vi "test图层(1)-原版.vi"() -> ()   [LabVIEW 2018]
doc: "This example demonstrates the use of binary morphological reconstruction in the particle analysis. The example allows you to keep the particles completely inside the ROI, completely outside the ROI or on the ROI."
uses:
  <vilib>/vision/NI_Vision_Development_Module.lvlib
panel:
  out "框&图层计数":dbl
  in  "Operation":T1(ring)
  out "Reconstructed Image":T2(plugin-control)
  out "Image":T2(plugin-control)
  in  "Stop":bool
  # "Overview: Demonstrate the use of the Binary Morphology Reconstruction feature of Vision Development Module.\nRequirements: Vision Development Module.\nInstructions:\n1. Run the VI.\n2. Select the ROI in which you want to filter the objects. Press the <Ctrl> key to select multiple ROIs. \n3. Choose the required \"Operation\".\n  - Inner particles: Keeps all the particles completely inside the ROI.\n  - Outer particles: Keeps the particles completely outside the ROI.\n  - Boundary particles: Keeps the particles which are touching the boundary."
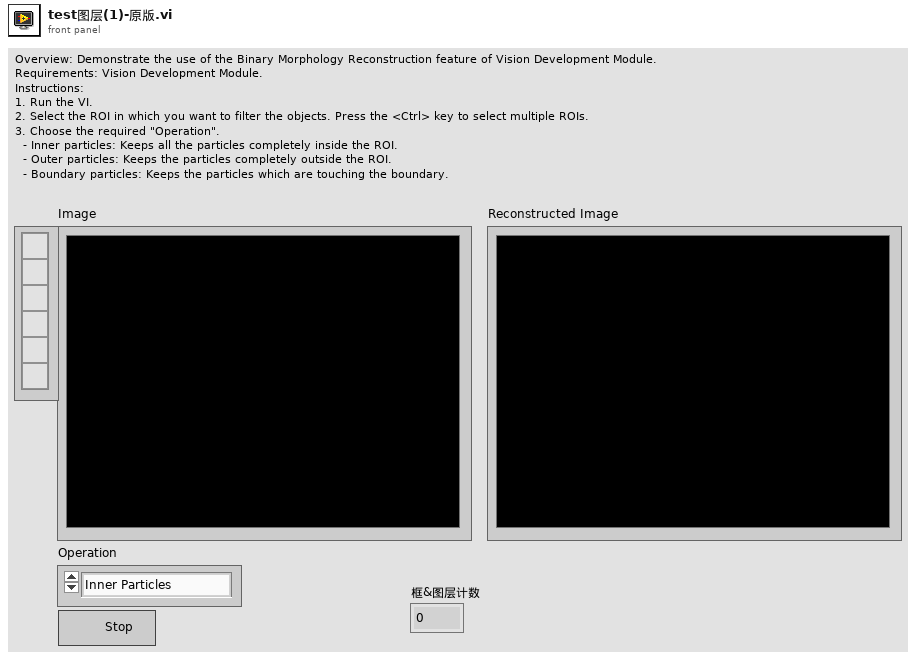
[diagram p1: front panel]
types:
  T1 = enum16{"Inner Particles", "Outer Particles", "Boundary Particles", "overlay rectangle"}
  T2 = typedef "IMAQ Image.ctl" = refnum<image>
  T3 = typedef "Image Type" = u32
  T4 = cluster{"Global Rectangle":i32[], "Contours":cluster{"Contour Type":u32, "ROI Type":u32, "Points":i32[]}[]}
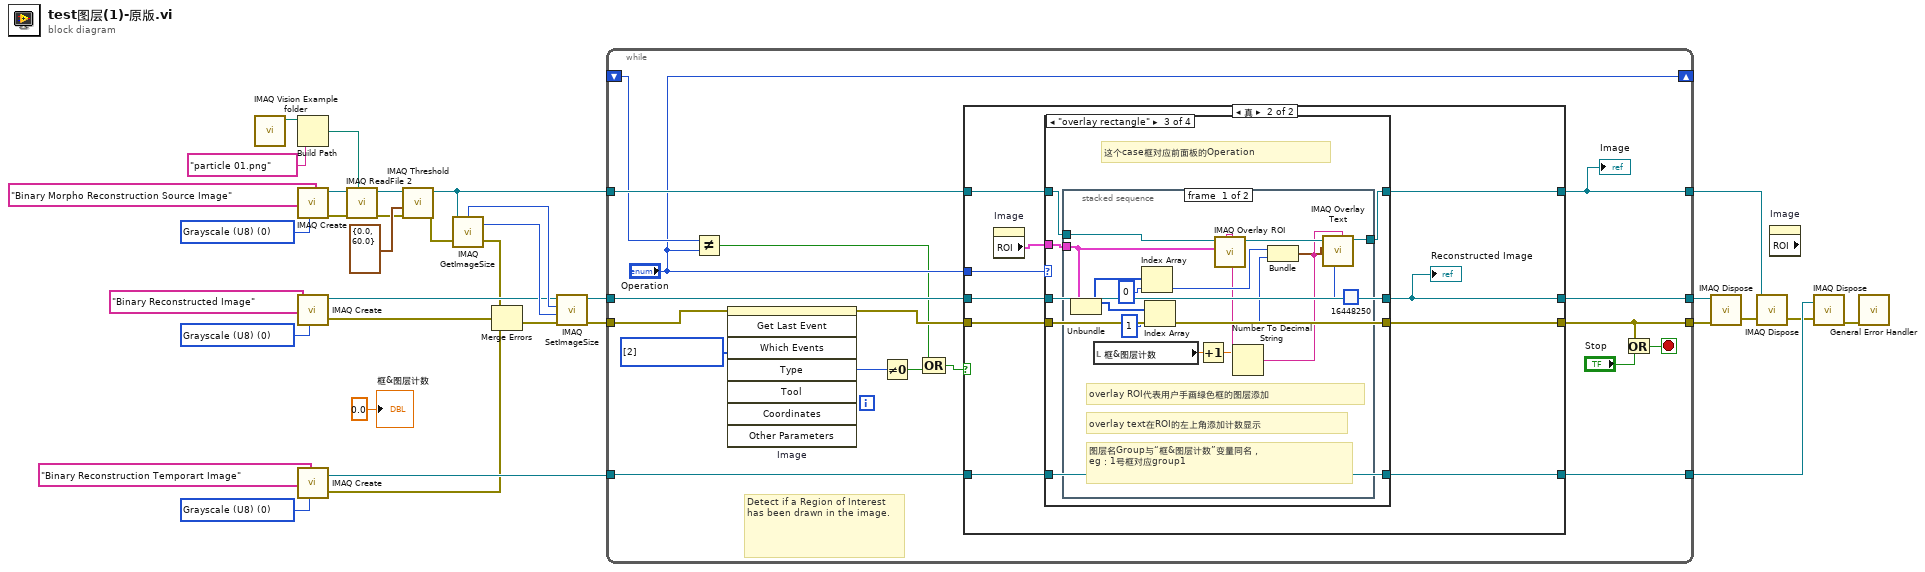
[diagram p0: block diagram]
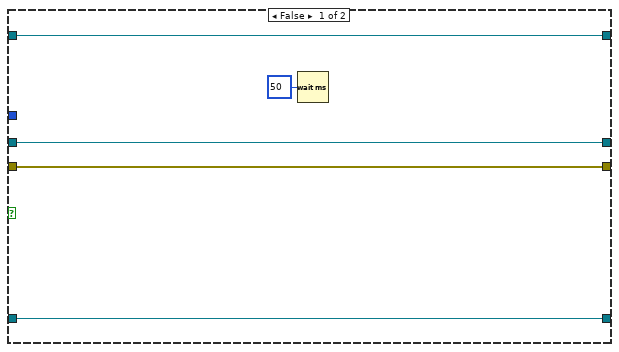
[diagram p2: hidden frame]
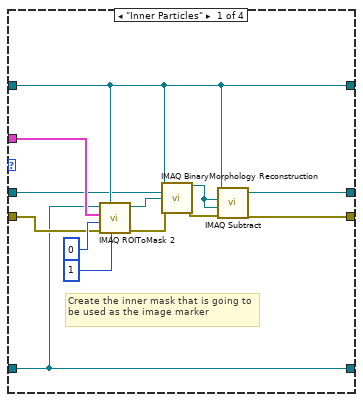
[diagram p3: hidden frame]
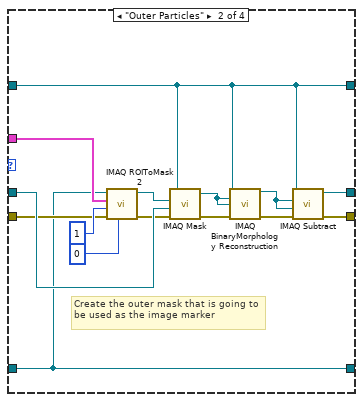
[diagram p4: hidden frame]
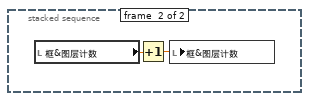
[diagram p5: hidden frame]
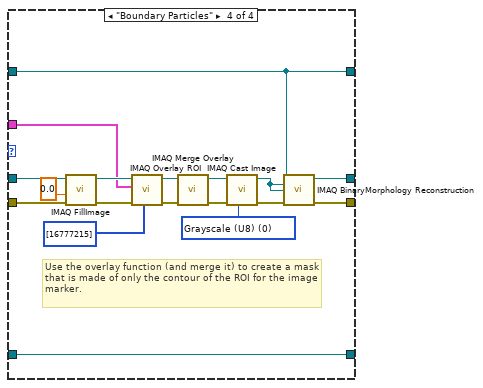
[diagram p6: hidden frame]
diagram:
  w24 = T3 0 items=["Grayscale (U8)", "Grayscale (I16)", "Grayscale (SGL)", "Complex (CSG)", "RGB (U32)", "HSL (U32)", "RGB (U64)", "Grayscale (U16)"] ("Image Type")
  w26 = T3 0 items=["Grayscale (U8)", "Grayscale (I16)", "Grayscale (SGL)", "Complex (CSG)", "RGB (U32)", "HSL (U32)", "RGB (U64)", "Grayscale (U16)"] ("Image Type")
  w27 = T3 0 items=["Grayscale (U8)", "Grayscale (I16)", "Grayscale (SGL)", "Complex (CSG)", "RGB (U32)", "HSL (U32)", "RGB (U64)", "Grayscale (U16)"] ("Image Type")
  n1 = call "IMAQ Vision Example folder.vi"() -> ("Example Image Path"=w33:path)  [unwired: 11 in]
  n2 = Build Path(base path=w33, name or relative path="particle 01.png") -> (appended path=w3:path)
  n3 = call "IMAQ Create"("Image Name"="Binary Morpho Reconstruction Source Image", "Image Type"=w26) -> ("New Image"=w30:T2, "error out"=w16:errorcluster)  [unwired: 2 in, 1 out]
  n4 = call "IMAQ Create"("Image Name"="Binary Reconstructed Image", "Image Type"=w27) -> ("New Image"=w20:T2, "error out"=w13:errorcluster)  [unwired: 2 in, 1 out]
  n5 = call "IMAQ Create"("Image Name"="Binary Reconstruction Temporart Image", "Image Type"=w24) -> ("New Image"=w21:T2, "error out"=w12:errorcluster)  [unwired: 2 in, 1 out]
  n6 = call "IMAQ ReadFile 2"("File Path"=w3, "error in (no error)"=w16, "Image"=w30) -> ("error out"=w15:errorcluster, "Image Out"=w18:T2)  [unwired: 4 in, 3 out]
  n7 = call "IMAQ Threshold"("error in (no error)"=w15, "Range"=cluster{"Lower value":sgl, "Upper value":sgl} {"Lower value"=0.0, "Upper value"=60.0}, "Image Src"=w18) -> ("error out"=w14:errorcluster, "Image Dst Out"=w2:T2)  [unwired: 3 in, 4 out]
  n8 = call "IMAQ GetImageSize"("Image"=w2, "error in (no error)"=w14) -> ("Y Resolution"=w22:i32, "X Resolution"=w23:i32, "error out"=w9:errorcluster)  [unwired: 2 out]
  n9 = Merge Errors(w9, w13, w12) -> (w11:errorcluster)
  n10 = call "IMAQ SetImageSize"("error in (no error)"=w11, "Y Resolution"=w22, "X Resolution"=w23, "Image"=w20) -> ("error out"=w10:errorcluster, "Image Out"=w19:T2)  [unwired: 1 out]
  n11 = while {
    tunnel: w2 -> [w52]
    tunnel: w19 -> [w51]
    tunnel: [w50] -> w29
    tunnel: [w35] -> w28
    tunnel: w21 -> [w49]
    shift-right: ["Operation"] -> _
    shift-left: _ -> [w48]
    tunnel: w10 -> [w44]
    tunnel: [w38] -> w7
    tunnel: [w42] -> w8
    stop <- w36 stop-if-true
    w45 = i32[] [2] items=["No Event"=0, "Click Event"=1, "Draw Event"=2, "Size Event"=4, "Scroll Event"=5, "Double Click Event"=8] ("Which Events")
    # "Detect if a Region of Interest has been drawn in the image."
    n12 = Not Equal?(x=w48, y="Operation") -> (x != y?=w41:bool)
    n13 = invoke on="Image" class="ImageControl" method="Get Last Event"(error in=w44, "Which Events"=w45) -> (error out=w43:errorcluster, "Type"=w46:i32)  [unwired: 6 in, 6 out]
    n14 = Not Equal To 0?(x=w46) -> (x != 0?=w40:bool)
    n15 = Compound Arithmetic op=OR(w41, w40) -> (w39:bool)
    n16 = case shown="真" w39 {
      tunnel: w52 -> [w57 w67]
      tunnel: w51 -> [w56 w66]
      tunnel: [w56 w65] -> w50
      tunnel: [w57 w64] -> w35
      tunnel: w49 -> [w54 w59]
      tunnel: "Operation" -> [_ w62]
      tunnel: w43 -> [w55 w61]
      tunnel: [w55 w60] -> w38
      tunnel: [w54 w58] -> w42
      frame False {
        n17 = Wait (ms)(milliseconds to wait=u32 50) -> ()  [unwired: 1 out]
      }
      frame True {
        n18 = property on="Image" class="ImageControl"() -> ("ROI"=w63:T4)  [unwired: 2 in, 2 out]
        n19 = case shown="\"overlay rectangle\"" w62 {
          tunnel: w67 -> [w75 w87 w98 w132]
          tunnel: w66 -> [w73 w88 w101 w124]
          tunnel: w59 -> [w68 w81 w99 w133]
          tunnel: [w77 w90 w101 w135] -> w65
          tunnel: w63 -> [w76 w89 w96 w125]
          tunnel: [w75 w87 w97 w132] -> w64
          tunnel: w61 -> [w72 w86 w100 w123]
          tunnel: [w69 w82 w100 w134] -> w60
          tunnel: [w68 w81 w99 w133] -> w58
          frame "Inner Particles" {
            # "Create the inner mask that is going to be used as the image marker"
            n20 = call "IMAQ ROIToMask 2"("Background Value (0)"=1, "Image Model"=w75, "error in (no error)"=w72, "Filling Value (255)"=0, "ROI Descriptor"=w76, "Image"=w68) -> ("error out"=w71:errorcluster, "Image Out"=w74:T2)  [unwired: 4 out]
            n21 = call "IMAQ BinaryMorphology Reconstruction"("Image Src"=w75, "Image Dst"=w73, "Image Marker"=w74, "error in (no error)"=w71) -> ("Image Dst Out"=w78:T2, "error out"=w70:errorcluster)  [unwired: 4 in, 6 out]
            n22 = call "IMAQ Subtract"("Image Src A"=w75, "Image Dst"=w78, "Image Src B"=w78, "error in (no error)"=w70) -> ("Image Dst Out"=w77:T2, "error out"=w69:errorcluster)  [unwired: 1 in, 2 out]
          }
          frame "Outer Particles" {
            # "Create the outer mask that is going to be used as the image marker"
            n23 = call "IMAQ ROIToMask 2"("Background Value (0)"=0, "error in (no error)"=w86, "Filling Value (255)"=1, "ROI Descriptor"=w89, "Image"=w81) -> ("error out"=w85:errorcluster, "Image Out"=w93:T2)  [unwired: 1 in, 4 out]
            n24 = call "IMAQ Mask"("error in (no error)"=w85, "Image Dst"=w88, "Image Mask"=w93, "Image Src"=w87) -> ("error out"=w84:errorcluster, "Image Dst Out"=w92:T2)  [unwired: 1 out]
            n25 = call "IMAQ BinaryMorphology Reconstruction"("Image Src"=w87, "Image Dst"=w92, "Image Marker"=w92, "error in (no error)"=w84) -> ("Image Dst Out"=w91:T2, "error out"=w83:errorcluster)  [unwired: 4 in, 6 out]
            n26 = call "IMAQ Subtract"("Image Src A"=w87, "Image Dst"=w91, "Image Src B"=w91, "error in (no error)"=w83) -> ("Image Dst Out"=w90:T2, "error out"=w82:errorcluster)  [unwired: 1 in, 2 out]
          }
          frame "overlay rectangle" {
            # "这个case框对应前面板的Operation"
            n27 = stacked-sequence {
              tunnel: w98 -> [w115 _]
              tunnel: [w113 _] -> w97
              tunnel: w96 -> [w112 _]
              frame #0 {
                # "图层名Group与“框&图层计数”变量同名，\neg：1号框对应group1"
                # "overlay text在ROI的左上角添加计数显示"
                # "overlay ROI代表用户手画绿色框的图层添加"
                n28 = Unbundle(w112) -> ("Global Rectangle"=w109:i32[])  [unwired: 1 out]
                n29 = local read "框&图层计数"() -> (w104:dbl)
                n30 = Index Array(array=w109, index=0 ("索引")) -> (element=w108:i32)
                n31 = Index Array(array=w109, index=1 ("索引")) -> (element=w107:i32)
                n32 = Increment(x=w104) -> (x+1=w102:dbl)
                n33 = Number To Decimal String(number=w102) -> (decimal integer string=w103:string)  [unwired: 1 in]
                n34 = call "IMAQ Overlay ROI"("Group"=w103, "ROI Descriptor"=w112, "Image"=w115) -> ("Image Out"=w114:T2)  [unwired: 7 in, 1 out]
                n35 = Bundle(w108, w107) -> (w106:cluster{i32, i32})  [unwired: 1 in]
                n36 = call "IMAQ Overlay Text"("Group"=w103, "Text Color (black)"=u32 16448250, "String"=w103, "Origin"=w106, "Image"=w114) -> ("Image Out"=w113:T2)  [unwired: 5 in, 1 out]
              }
              frame #1 {
                n37 = local read "框&图层计数"() -> (w117:dbl)
                n38 = Increment(x=w117) -> (x+1=w116:dbl)
                n39 = local write "框&图层计数"(w116) -> ()
              }
            }
          }
          frame "Boundary Particles" {
            w127 = T3 0 items=["Grayscale (U8)", "Grayscale (I16)", "Grayscale (SGL)", "Complex (CSG)", "RGB (U32)", "HSL (U32)", "RGB (U64)", "Grayscale (U16)"] ("Image Type")
            # "Use the overlay function (and merge it) to create a mask that is made of only the contour of the ROI for the image marker."
            n40 = call "IMAQ FillImage"("error in (no error)"=w123, "Pixel Value (U8, U16, I16, Float)"=sgl 0.0, "Image"=w124) -> ("error out"=w122:errorcluster, "Image Out"=w130:T2)  [unwired: 4 in, 3 out]
            n41 = call "IMAQ Overlay ROI"("Colors (Green)"=u32[] [16777215], "error in (no error)"=w122, "ROI Descriptor"=w125, "Image"=w130) -> ("error out"=w121:errorcluster, "Image Out"=w131:T2)  [unwired: 2 in, 4 out]
            n42 = call "IMAQ Merge Overlay"("error in (no error)"=w121, "Image Src"=w131) -> ("error out"=w120:errorcluster, "Image Dst Out"=w128:T2)  [unwired: 3 in, 5 out]
            n43 = call "IMAQ Cast Image"("Image Type"=w127, "error in (no error)"=w120, "Image Src"=w128) -> ("error out"=w119:errorcluster, "Image Dst Out"=w118:T2)  [unwired: 3 in, 4 out]
            n44 = call "IMAQ BinaryMorphology Reconstruction"("Image Src"=w132, "Image Dst"=w118, "Image Marker"=w118, "error in (no error)"=w119) -> ("Image Dst Out"=w135:T2, "error out"=w134:errorcluster)  [unwired: 4 in, 6 out]
          }
        }
        "Reconstructed Image" <- w65
      }
    }
    "Image" <- w35
    n45 = Or(x=w38, y="Stop") -> (x .or. y?=w36:bool)
  }
  n46 = call "IMAQ Dispose"("Image"=w29, "error in (no error)"=w7) -> ("error out"=w6:errorcluster)  [unwired: 1 in, 3 out]
  n47 = call "IMAQ Dispose"("Image"=w28, "error in (no error)"=w6) -> ("error out"=w5:errorcluster)  [unwired: 1 in, 3 out]
  n48 = property on="Image" class="ImageControl" props=["ROI"]() -> ()  [unwired: 2 in, 3 out]
  n49 = call "IMAQ Dispose"("Image"=w8, "error in (no error)"=w5) -> ("error out"=w4:errorcluster)  [unwired: 1 in, 3 out]
  n50 = call <vilib>:"General Error Handler.vi"("error in (no error)"=w4) -> ()  [unwired: 10 in, 5 out]
  "框&图层计数" <- 0.0 ("数值")
